vi "BIOS Info.vi"() -> ()   [LabVIEW 2013]
uses:
  System.Management
panel:
  out "Table Control":string[][](table)=[["Dell Inc.                "], ["Phoenix ROM BIOS PLUS Version 1.10 2.6.0 "], [""], ["2.6.0 "], ["DELL   - 15"]]
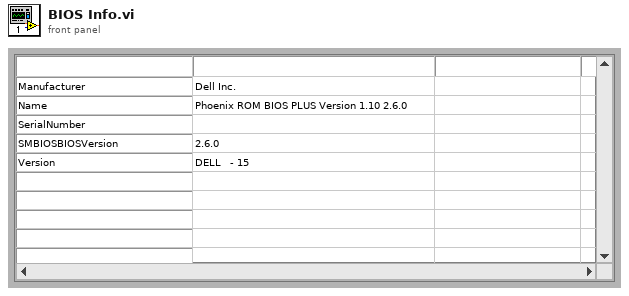
[diagram p1: front panel]
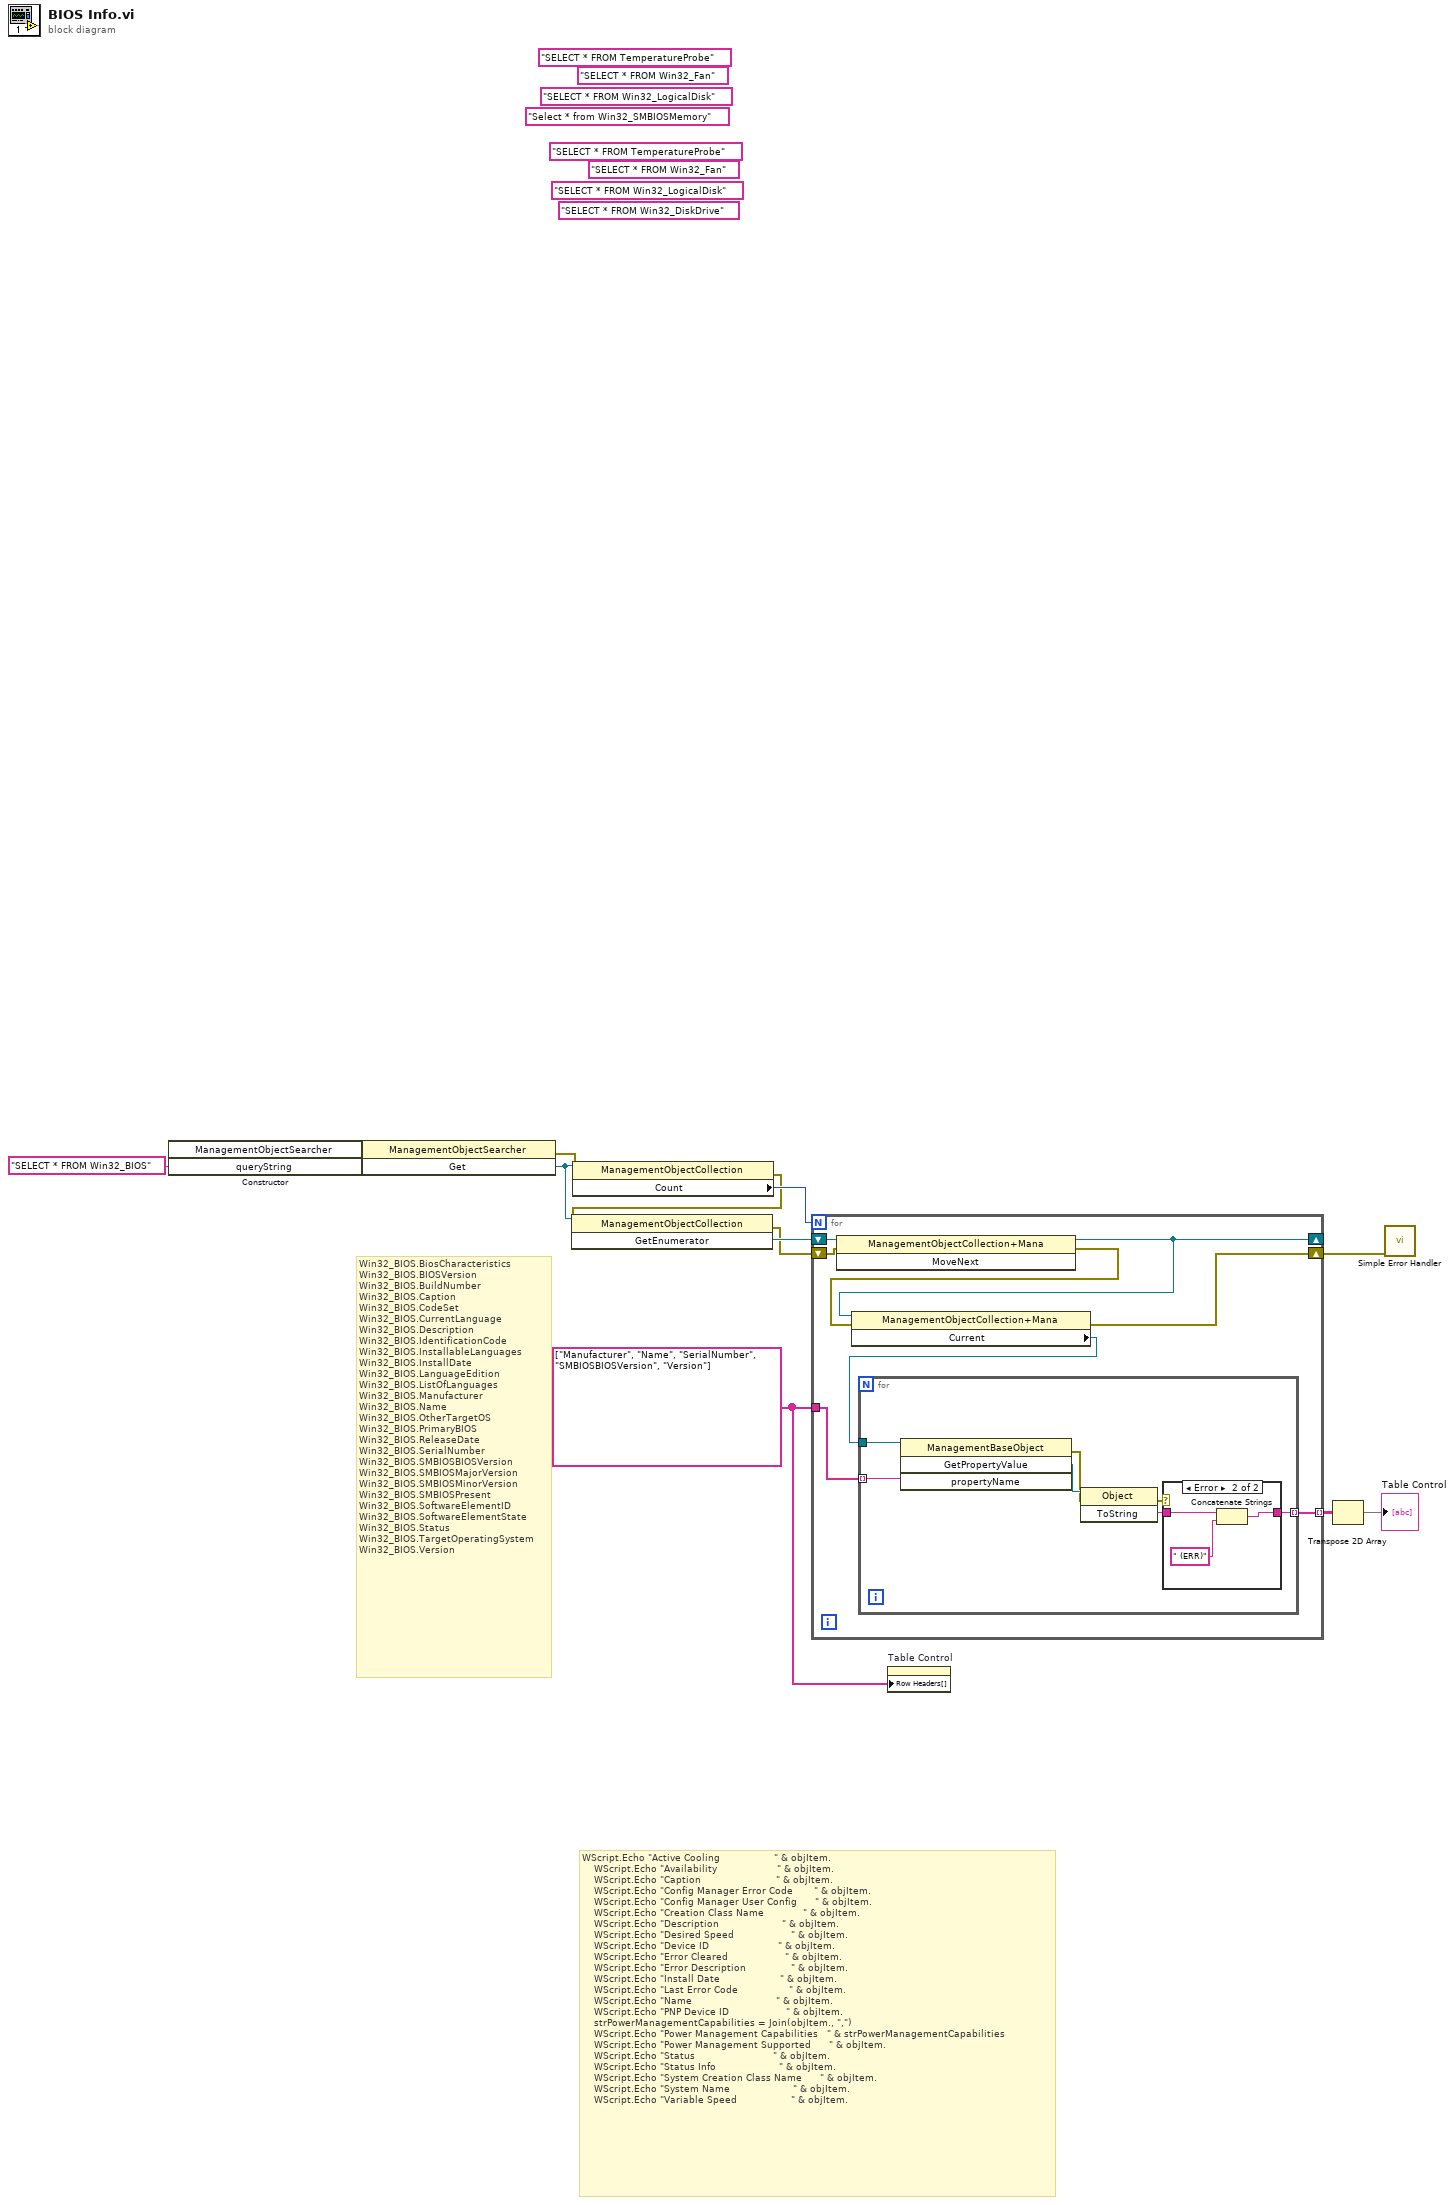
[diagram p0: block diagram]
diagram:
  w4 = string[] ["Manufacturer", "Name", "SerialNumber", "SMBIOSBIOSVersion", "Version"]
  (unwired) "SELECT * FROM Win32_LogicalDisk" ("queryString")
  (unwired) "SELECT * FROM Win32_Fan" ("queryString")
  (unwired) "Select * from Win32_SMBIOSMemory" ("queryString")
  (unwired) "SELECT * FROM TemperatureProbe" ("queryString")
  (unwired) "SELECT * FROM Win32_LogicalDisk" ("queryString")
  (unwired) "SELECT * FROM Win32_Fan" ("queryString")
  (unwired) "SELECT * FROM Win32_DiskDrive" ("queryString")
  (unwired) "SELECT * FROM TemperatureProbe" ("queryString")
  # "Win32_BIOS.BiosCharacteristics\nWin32_BIOS.BIOSVersion\nWin32_BIOS.BuildNumber\nWin32_BIOS.Caption\nWin32_BIOS.CodeSet\nWin32_BIOS.CurrentLanguage\nWin32_BIOS.Description\nWin32_BIOS.IdentificationCode\nWin32_BIOS.InstallableLanguages\nWin32_BIOS.InstallDate\nWin32_BIOS.LanguageEdition\nWin32_BIOS.ListOfLanguages\nWin32_BIOS.Manufacturer\nWin32_BIOS.Name\nWin32_BIOS.OtherTargetOS\nWin32_BIOS.PrimaryBIOS\nWin32_BIOS.ReleaseDate\nWin32_BIOS.SerialNumber\nWin32_BIOS.SMBIOSBIOSVersion\nWin32_BIOS.SMBIOSMajorVersion\nWin32_BIOS.SMBIOSMinorVersion\nWin32_BIOS.SMBIOSPresent\nWin32_BIOS.SoftwareElementID\nWin32_BIOS.SoftwareElementState\nWin32_BIOS.Status\nWin32_BIOS.TargetOperatingSystem\nWin32_BIOS.Version"
  # "WScript.Echo \"Active Cooling                  \" & objItem. \n    WScript.Echo \"Availability                    \" & objItem. \n    WScript.Echo \"Caption                         \" & objItem. \n    WScript.Echo \"Config Manager Error Code       \" & objItem. \n    WScript.Echo \"Config Manager User Config      \" & objItem. \n    WScript.Echo \"Creation Class Name             \" & objItem. \n    WScript.Echo \"Description                     \" & objItem. \n    WScript.Echo \"Desired Speed                   \" & objItem. \n    WScript.Echo \"Device ID                       \" & objItem. \n    WScript.Echo \"Error Cleared                   \" & objItem. \n    WScript.Echo \"Error Description               \" & objItem. \n    WScript.Echo \"Install Date                    \" & objItem. \n    WScript.Echo \"Last Error Code                 \" & objItem. \n    WScript.Echo \"Name                            \" & objItem. \n    WScript.Echo \"PNP Device ID                   \" & objItem. \n    strPowerManagementCapabilities = Join(objItem., \",\") \n    WScript.Echo \"Power Management Capabilities   \" & strPowerManagementCapabilities \n    WScript.Echo \"Power Management Supported      \" & objItem. \n    WScript.Echo \"Status                          \" & objItem. \n    WScript.Echo \"Status Info                     \" & objItem. \n    WScript.Echo \"System Creation Class Name      \" & objItem. \n    WScript.Echo \"System Name                     \" & objItem. \n    WScript.Echo \"Variable Speed                  \" & objItem."
  n1 = constructor class="ManagementObjectSearcher"("queryString"="SELECT * FROM Win32_BIOS") -> (reference out=w11:refnum<k24>, error out=w9:errorcluster)  [unwired: 3 in, 2 out]
  n2 = invoke class="ManagementObjectSearcher" method="Get"(reference=w11, error in=w9) -> (error out=w10:errorcluster, "Get"=w12:refnum<k24>)  [unwired: 1 in, 1 out]
  n3 = property class="ManagementObjectCollection"(reference=w12, error in=w10) -> (error out=w3:errorcluster, "Count"=w13:i32)  [unwired: 1 out]
  n4 = invoke class="ManagementObjectCollection" method="GetEnumerator"(reference=w12, error in=w3) -> (error out=w2:errorcluster, "GetEnumerator"=w7:refnum<k24>)  [unwired: 1 in, 1 out]
  n5 = for {
    N: w13 -> [_]
    shift-right: [w20] -> _
    shift-left: w7 -> [w21]
    tunnel: [w19] -> w6 mode=indexing
    tunnel: w4 -> [w18]
    shift-right: [w14] -> w1
    shift-left: w2 -> [w16]
    n6 = invoke class="ManagementObjectCollection+Mana" method="MoveNext"(reference=w21, error in=w16) -> (reference out=w20:refnum<k24>, error out=w15:errorcluster)  [unwired: 1 in, 1 out]
    n7 = property class="ManagementObjectCollection+Mana"(reference=w20, error in=w15) -> (error out=w14:errorcluster, "Current"=w17:refnum<k24>)  [unwired: 1 out]
    n8 = for {
      tunnel: [w24] -> w19 mode=indexing
      tunnel: w17 -> [w26]
      tunnel: w18 -> [w25] mode=indexing
      n9 = invoke class="ManagementBaseObject" method="GetPropertyValue"(reference=w26, "propertyName"=w25) -> (error out=w27:errorcluster, "GetPropertyValue"=w28:refnum<k24>)  [unwired: 2 in, 2 out]
      n10 = invoke class="Object" method="ToString"(reference=w28, error in=w27) -> (error out=w22:errorcluster, "ToString"=w23:string)  [unwired: 1 in, 1 out]
      n11 = case shown="Error" w22 {
        tunnel: [w29 w30] -> w24
        tunnel: w23 -> [w29 w31]
        frame No Error {
        }
        frame Error {
          n12 = Concatenate Strings(w31, " (ERR)" ("string")) -> (w30:string)
        }
      }
    }
  }
  n13 = property on="Table Control" class="Tbl (strict)"("Row Headers[]"=w4) -> ()  [unwired: 2 in, 2 out]
  n14 = Transpose 2D Array(2D array=w6) -> (transposed array=→"Table Control":string[][])
  n15 = call <vilib>:"Simple Error Handler.vi"("error in (no error)"=w1) -> ()  [unwired: 1 in, 8 out]
